vi "Initialize.vi"(8 "error in (no error)":errorcluster, 9 "Reset? (T: Yes)":bool=TRUE, 10 "ID Query? (T: Yes)":bool=TRUE, 11 "VISA resource name":refnum<visa-resource-name>) -> (0 "error out":errorcluster, 3 "VISA resource name out":refnum<visa-resource-name>)   [LabVIEW 2020, in "LeCroy Wave Series.lvlib"]
doc: "Establishes communication with the instrument and optionally performs an instrument identification query and/or an instrument reset. It also places the instrument in a default state needed for other instrument driver operations. Therefore, call this VI before calling other instrument driver VIs for this instrument. Generally, you need to call the <B>Initialize VI</B> only once at the beginning of an application."
uses:
  LeCroy Wave Series.lvlib
panel:
  # "(c) 2008 - 2012 NATIONAL INSTRUMENTS.  ALL RIGHTS RESERVED."
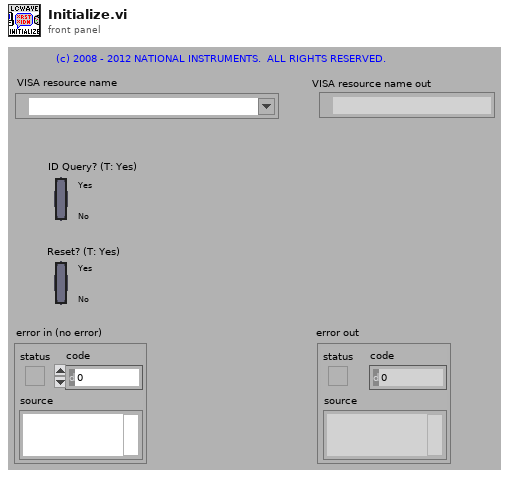
[diagram p1: front panel]
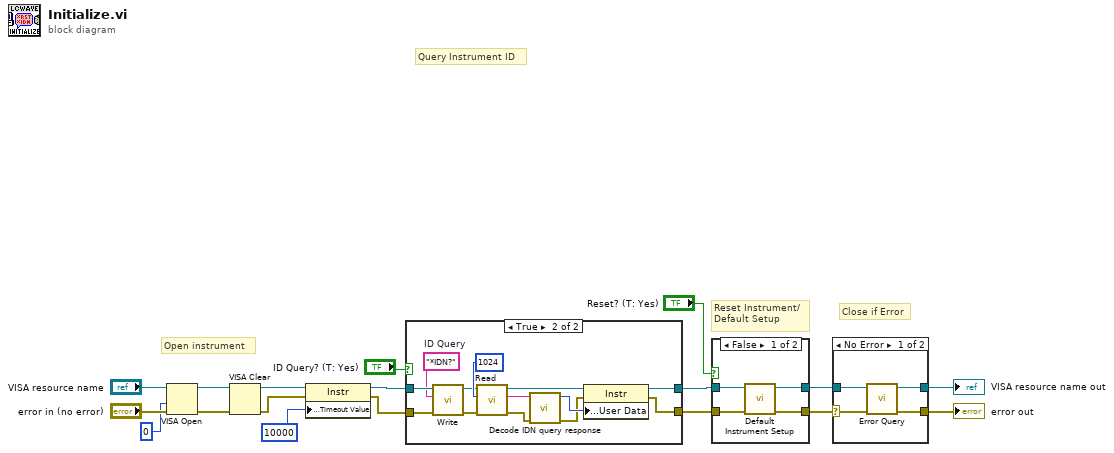
[diagram p0: block diagram]
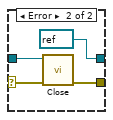
[diagram p2: hidden frame]
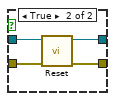
[diagram p3: hidden frame]
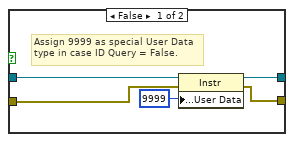
[diagram p4: hidden frame]
diagram:
  # "Close if Error"
  # "Query Instrument ID"
  # "Reset Instrument/\nDefault Setup"
  # "Open instrument"
  n1 = VISA Open(access mode=u32 0, error in (no error)="error in (no error)", VISA resource name="VISA resource name") -> (VISA resource name=w11:refnum<visa-resource-name>, error out=w10:errorcluster)  [unwired: 2 in]
  n2 = VISA Clear(VISA resource name=w11, error in (no error)=w10) -> (VISA resource name out=w9:refnum<visa-resource-name>, error out=w8:errorcluster)
  n3 = property on="Property Node" class="Instr"(reference=w9, error in=w8, "General Settings:Timeout Value"=u32 10000) -> (reference out=w3:refnum<visa-resource-name>, error out=w2:errorcluster)
  n4 = case shown="True" "ID Query? (T: Yes)" {
    tunnel: [w21 w25] -> w17
    tunnel: [w20 w29] -> w18
    tunnel: w3 -> [w23 w32]
    tunnel: w2 -> [w22 w33]
    frame False {
      # "Assign 9999 as special User Data\ntype in case ID Query = False."
      n5 = property on="Property Node" class="Instr"(reference=w23, error in=w22, "General Settings:User Data"=u32 9999) -> (reference out=w20:refnum<visa-resource-name>, error out=w21:errorcluster)
    }
    frame True {
      w31 = "*IDN?"  # ID Query
      n6 = call "Write.vi"("error in (no error)"=w33, "Write Buffer"=w31, "VISA resource name"=w32) -> ("error out"=w34:errorcluster, "VISA resource name out"=w35:refnum<visa-resource-name>)  [unwired: 6 in, 1 out]
      n7 = call "Read.vi"("error in (no error)"=w34, "Byte Count"=u32 1024, "VISA resource name"=w35) -> ("error out"=w27:errorcluster, "Read Buffer"=w24:string, "VISA resource name out"=w30:refnum<visa-resource-name>)  [unwired: 5 in, 1 out]
      n8 = call "Decode IDN query response.vi"("error in (no error)"=w27, "*IDN? result"=w24) -> ("error out"=w26:errorcluster, "Series ID"=w28:u32)  [unwired: 6 in, 2 out]
      n9 = property on="Property Node" class="Instr"(reference=w30, error in=w26, "General Settings:User Data"=w28) -> (reference out=w29:refnum<visa-resource-name>, error out=w25:errorcluster)
    }
  }
  n10 = case shown="False" "Reset? (T: Yes)" {
    tunnel: w17 -> [w39 w41]
    tunnel: [w38 w44] -> w4
    tunnel: w18 -> [w40 w42]
    tunnel: [w37 w43] -> w5
    frame False {
      n11 = call "Default Instrument Setup.vi"("error in (no error)"=w39, "VISA resource name"=w40) -> ("error out"=w38:errorcluster, "VISA resource name out"=w37:refnum<visa-resource-name>)  [unwired: 8 in]
    }
    frame True {
      n12 = call "Reset.vi"("error in (no error)"=w41, "VISA resource name"=w42) -> ("error out"=w44:errorcluster, "VISA resource name out"=w43:refnum<visa-resource-name>)  [unwired: 8 in]
    }
  }
  n13 = case shown="No Error" w4 {
    selector: w4 -> [w46 w50]
    tunnel: w5 -> [w45 w51]
    tunnel: [w48 refnum<visa-resource-name> refnum ("VISA resource name out")] -> w7
    tunnel: [w47 w52] -> w6
    frame No Error {
      n14 = call "Error Query.vi"("error in (no error)"=w46, "VISA resource name"=w45) -> ("error out"=w47:errorcluster, "VISA resource name out"=w48:refnum<visa-resource-name>)  [unwired: 6 in, 2 out]
    }
    frame Error {
      n15 = call "Close.vi"("error in (no error)"=w50, "VISA resource name"=w51) -> ("error out"=w52:errorcluster)  [unwired: 9 in]
    }
  }
  "VISA resource name out" <- w7
  "error out" <- w6
